vi "Get_CCD_temperature_setpoint.vi"(8 "error in":errorcluster, 11 "camera handle in":u64) -> (0 "error out":errorcluster, 1 "temperature setpoint (C)":dbl, 3 "camera handle out":u64)   [LabVIEW 2014, in "PICam.lvlib"]
doc: "Reads the current temperature setpoint in Celsius."
uses:
  PICam.lvlib
  Program Files/Princeton Instruments/PICam/Runtime/Picam32.dll
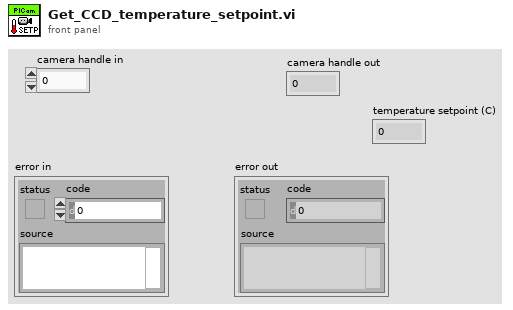
[diagram p1: front panel]
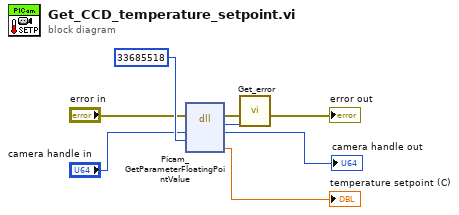
[diagram p0: block diagram]
diagram:
  n1 = dll-call lib="C:/Program Files/Princeton Instruments/PICam/Runtime/Picam32.dll" fn="Picam_GetParameterFloatingPointValue"(error in="error in", "camera"="camera handle in", "PicamParameter"=u32 33685518) -> (error out=w8:errorcluster, "return type"=w7:i32, "camera"=→"camera handle out":u64, "temperature"=→"temperature setpoint (C)":dbl)  [unwired: 4 in, 1 out]
  n2 = call "Get_error.vi"("PICam_Error"=w7, "error in (no error)"=w8) -> ("error out"=→"error out":errorcluster)  [unwired: 9 in]
